vi "ExSubOpenSpect.vi"(0 "error in (no error)":errorcluster) -> (1 "Spectromete Handle":u32, 2 "error out":errorcluster)   [LabVIEW 2010]
uses:
  GlobalSpectHdl.vi
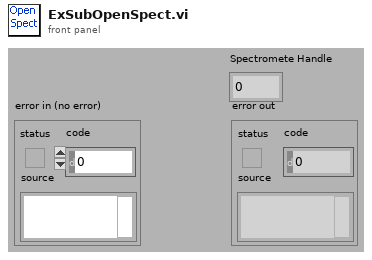
[diagram p1: front panel]
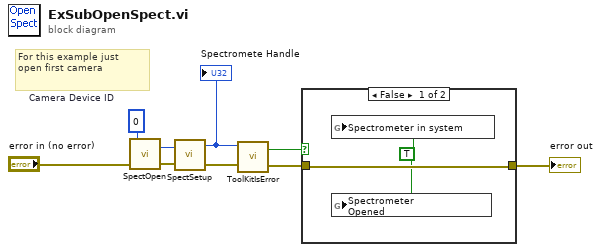
[diagram p0: block diagram]
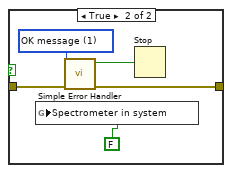
[diagram p2: hidden frame]
diagram:
  w5 = u32 0  # Camera Device ID
  # "For this example just\nopen first camera"
  n1 = call <userlib>:"SpectOpen.vi"("error in"="error in (no error)", "Spectrometer ID"=w5) -> ("error out"=w3:errorcluster, "Spectrometer Handle"=w4:u32)  [unwired: 1 in]
  n2 = call <userlib>:"SpectSetup.vi"("error in"=w3, "Spectrometer Handle"=w4) -> ("error out"=w2:errorcluster, "Spectrometer Handle"=w1:u32)
  "Spectromete Handle" <- w1
  n3 = call <userlib>:"ToolKitIsError.vi"("error in"=w2, "Reserved"=w1) -> ("error out"=w8:errorcluster, "Error Flag"=w9:bool)
  n4 = case shown="False" w9 {
    tunnel: w8 -> [w11 w16]
    tunnel: [w11 w14] -> w7
    frame False {
      w10 = TRUE
      n5 = global write "GlobalSpectHdl.vi" "Spectrometer in system"(w10) -> ()
      n6 = global write "GlobalSpectHdl.vi" "Spectrometer \nOpened"(w10) -> ()
    }
    frame True {
      w13 = u16 1 items=["no dialog", "OK message", "continue or stop message"] ("type of dialog (OK msg:1)")
      n7 = global write "GlobalSpectHdl.vi" "Spectrometer in system"(FALSE) -> ()
      n8 = call <vilib>:"Simple Error Handler.vi"("type of dialog (OK msg:1)"=w13, "error in (no error)"=w16) -> ("error?"=w15:bool, "error out"=w14:errorcluster)  [unwired: 3 in, 3 out]
      n9 = Stop(stop? (T)=w15) -> ()
    }
  }
  "error out" <- w7
